vi "pressure system controller v13 MEMStoGO (old) 2015.vi"() -> ()   [LabVIEW 2015]
uses:
  <vilib>/DAQmx/write.llb/DAQmx Write (Digital 1D Bool 1Chan 1Samp).vi
  <vilib>/DAQmx/write.llb/DAQmx Write (Analog DBL 1Chan 1Samp).vi
  <vilib>/DAQmx/read.llb/DAQmx Read (Analog DBL 1Chan 1Samp).vi
  <vilib>/DAQmx/create/channels.llb/DAQmx Create Channel (DO-Digital Output).vi
  <vilib>/DAQmx/miscellaneous.llb/DAQmx Fill In Error Info.vi
  <vilib>/DAQmx/create/channels.llb/DAQmx Create Channel (AI-Voltage-Basic).vi
  <vilib>/DAQmx/configure/timing.llb/DAQmx Timing (Sample Clock).vi
  <vilib>/DAQmx/create/channels.llb/DAQmx Create Channel (AO-Current-Basic).vi
  <vilib>/express/express shared/transition.llb/Dynamic To Waveform Array.vi
  <vilib>/express/express signal manip/GetorSetDDTAttributes/Set DDT Attributes/SetT0.vi
  <vilib>/express/express shared/transition.llb/Waveform Array To Dynamic.vi
  <instrlib>/Keithley 24XX/Public/Data/Read (Single Point).vi
  <vilib>/express/express signal manip/GetorSetDDTAttributes/Set DDT Attributes/Set DDT Properties.xnode
  <vilib>/ptbypt/NI_PtbyPt.lvlib
  <instrlib>/Keithley 24XX/Keithley 24XX.lvlib
  <instrlib>/Agilent E4980/Agilent E4980.lvlib
panel:
  in  "MUX4: Keithley (-)":T1(radio)
  in  "MUX3: Keithley (+)":T1(radio)
  in  "MUX2: LCR (-)":T1(radio)
  in  "MUX1: LCR (+)":T1(radio)
  in  "Write to file":bool=TRUE caption="Enable"
  out "Pressure":dbl
  in  "Turn on (MAKE SURE TURN OFF)":bool=TRUE
  out "Impedance":dbl format="%^#_6e"
  out "Phase (deg)":dbl
  in  "Function (0: Cp-D)":u16(ring)=17 items=["Cp-D", "Cp-Q", "Cp-G", "Cp-Rp", "Cs-D", "Cs-Q", "Cs-Rs", "Lp-D", "Lp-Q", "Lp-G", "Lp-Rp", "Lp-Rdc", "Ls-D", "Ls-Q", "Ls-Rs", "Ls-Rdc", "R-X", "Z-thd", "Z-thr", "G-B", "Y-thd", "Y-thr", "Vdc-Idc"]
  in  "Signal Level (1.0 V)":dbl=1.0
  in  "Averaging Factor (1)":i32=1
  in  "Measurement Time (1: Medium)":u16(ring) items=["Short", "Medium", "Long"]
  in  "Signal Frequency":dbl=10000.0
  out "Resistance (Mohm)":dbl
  out "Current (uA)":sgl
  out "Voltage":sgl
  in  "Loop sample rate (samples per second)":dbl=5.0
  in  "Current duration (s)":dbl=2.0
  out "Time Counter":i32
  in  "Keithley Output (uA)":dbl=1.0
  in  "Compliance (V)":dbl=21.0
  in  "Inject Current":bool
  out "Supply Current":dbl
  in  "Set Point Pressure (mmHg)":dbl min=0.0 max=500.0
  in  "stop":bool
  # "Switch"
  # "Keithley Settings"
  # "Pressure Setup"
  # "LCR Settings"
  # "1KHz for water"
  # "MAX: 500"
  # "10KHz for PBS"
  # "seconds"
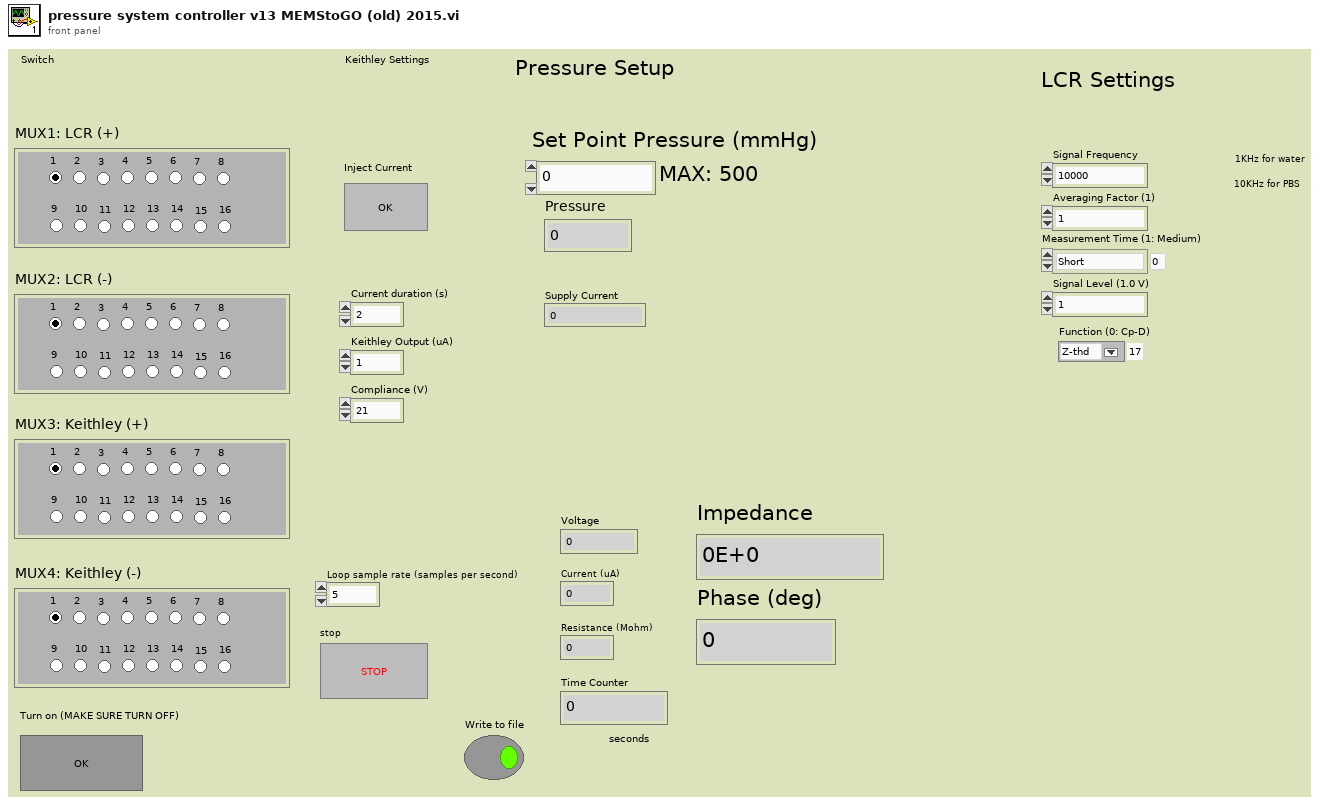
[diagram p1: front panel]
types:
  T1 = enum32{"1", "2", "3", "4", "5", "6", "7", "8", "9", "10", "11", "12", "13", "14", "15", "16"}
  T2 = cluster{"Primary Parameter":dbl, "Secondary Parameter":dbl}
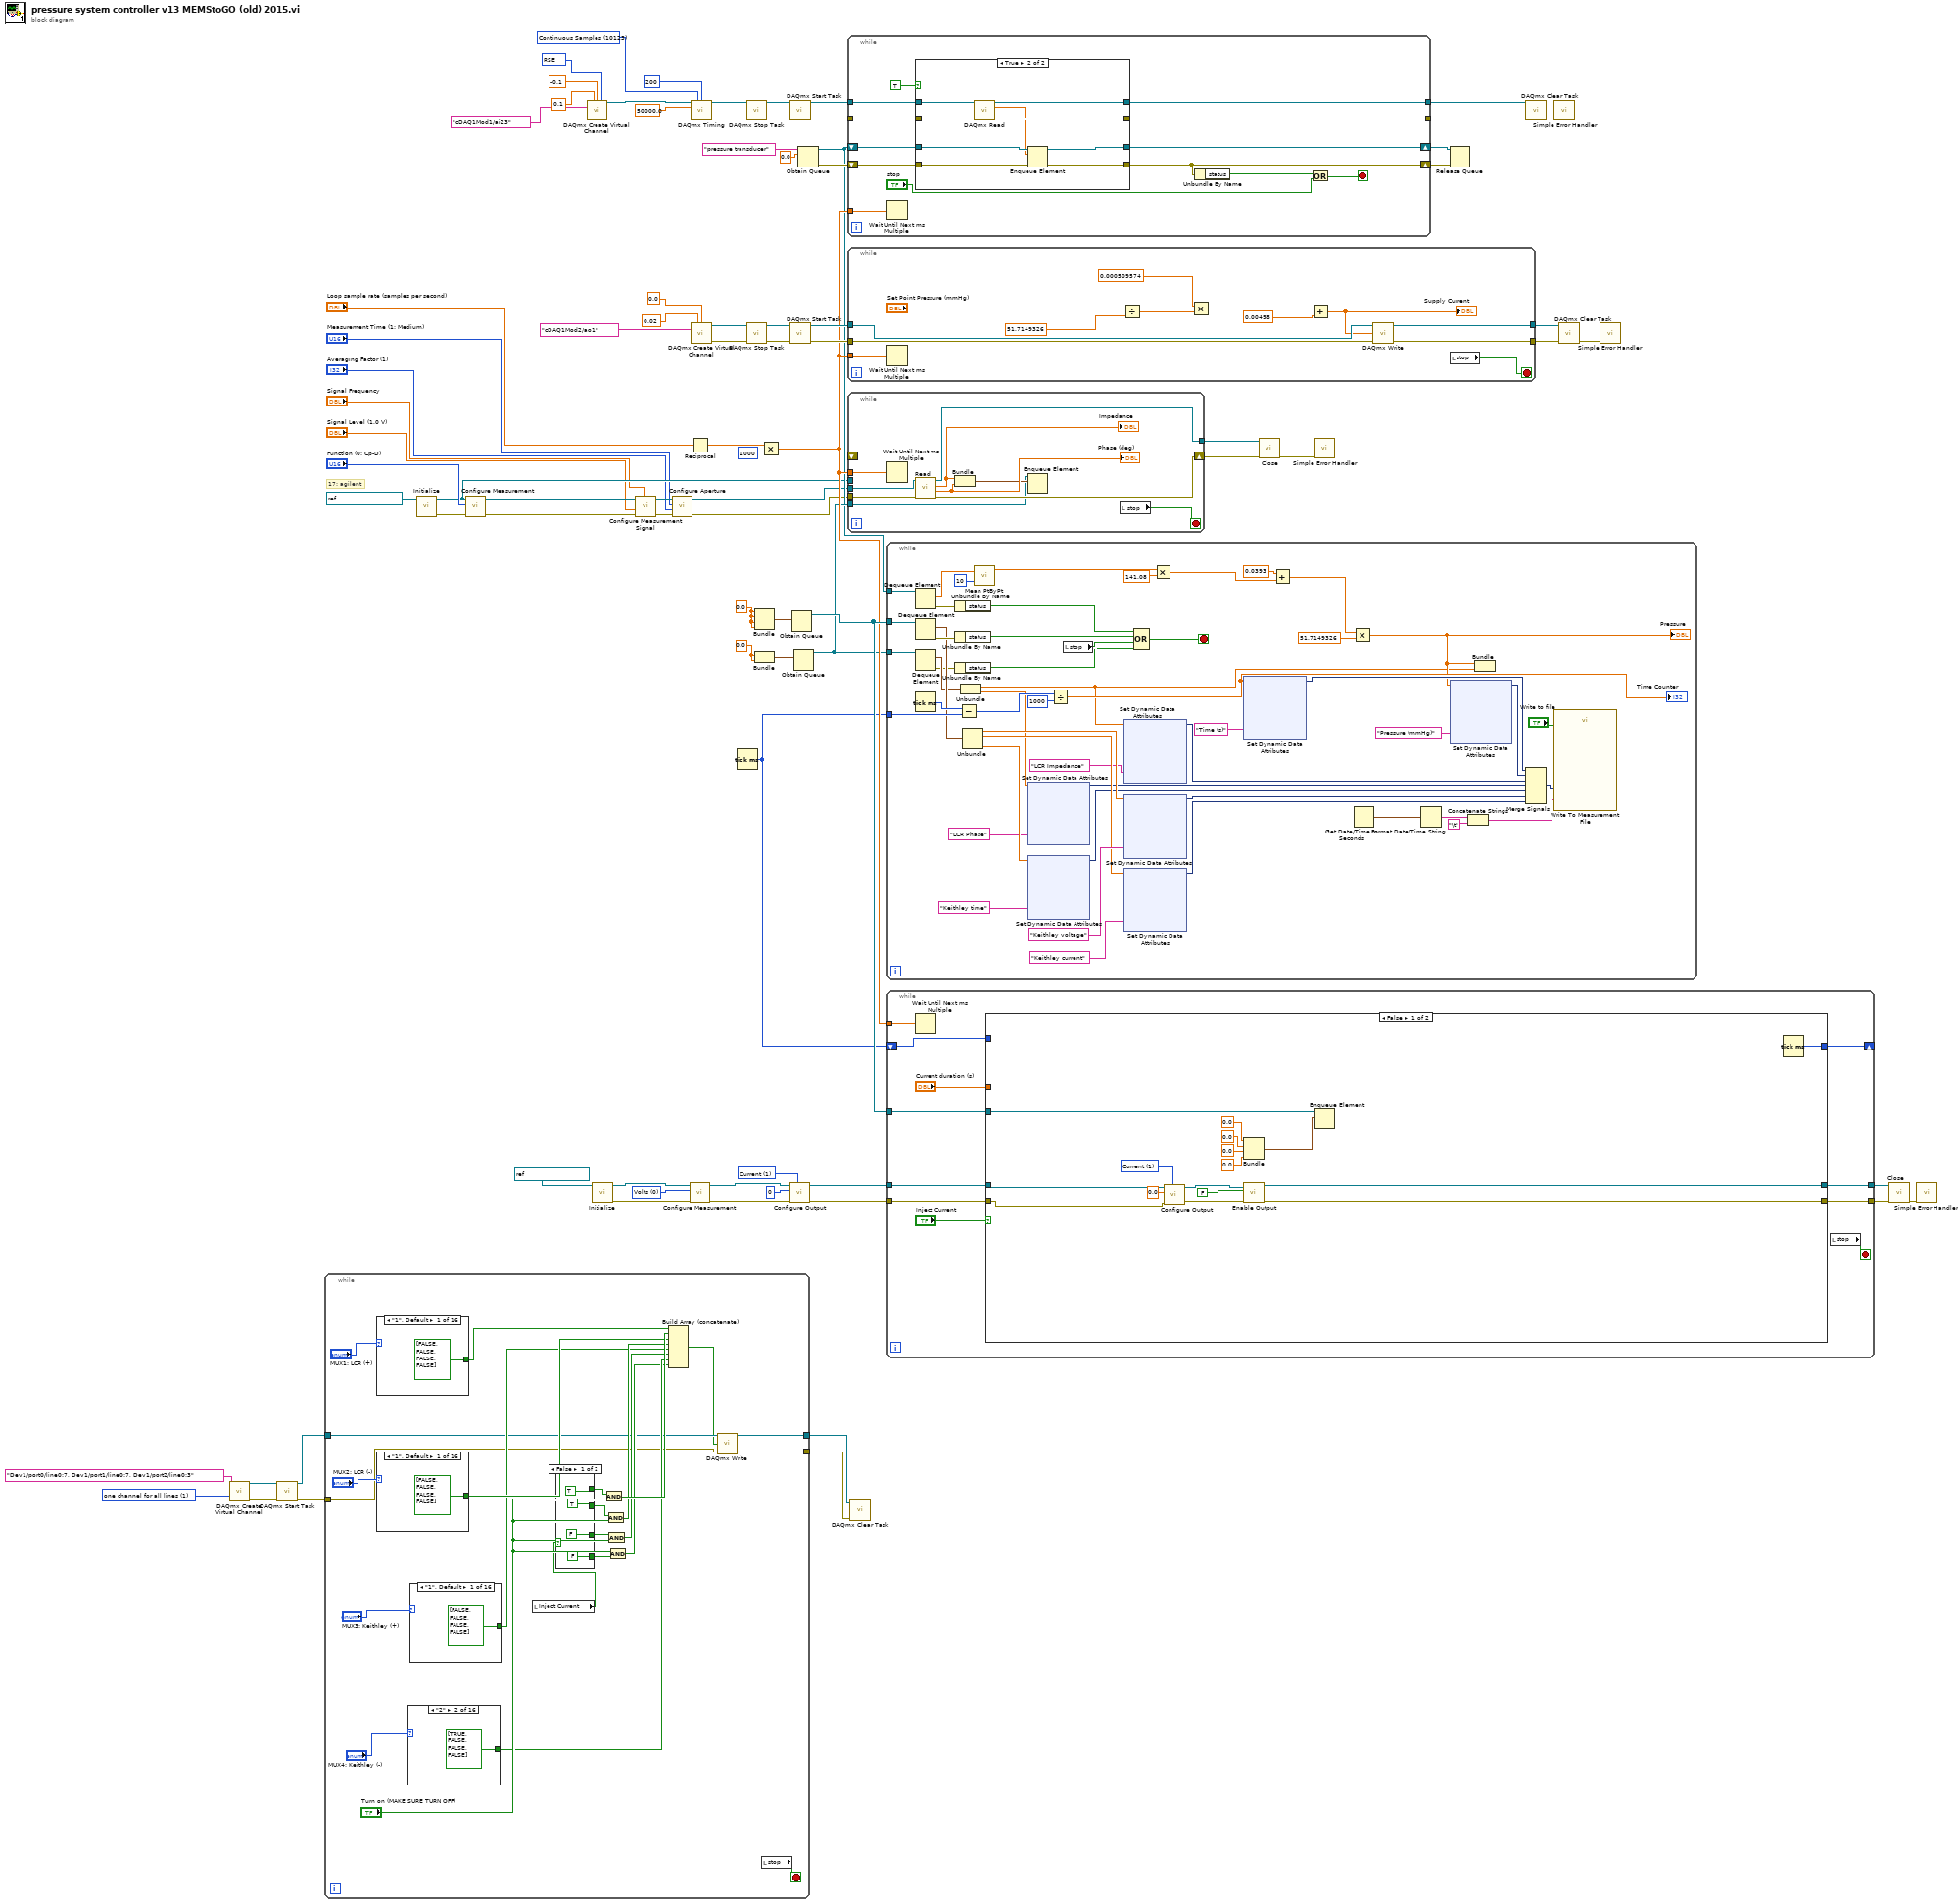
[diagram p0: block diagram]
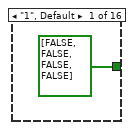
[diagram p2: hidden frame]
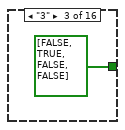
[diagram p3: hidden frame]
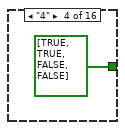
[diagram p4: hidden frame]
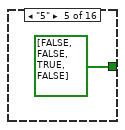
[diagram p5: hidden frame]
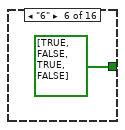
[diagram p6: hidden frame]
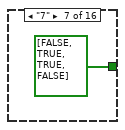
[diagram p7: hidden frame]
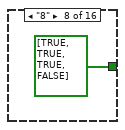
[diagram p8: hidden frame]
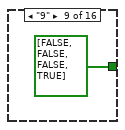
[diagram p9: hidden frame]
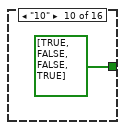
[diagram p10: hidden frame]
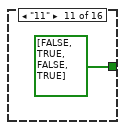
[diagram p11: hidden frame]
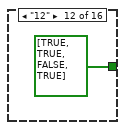
[diagram p12: hidden frame]
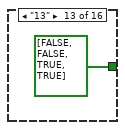
[diagram p13: hidden frame]
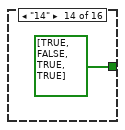
[diagram p14: hidden frame]
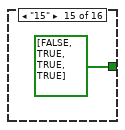
[diagram p15: hidden frame]
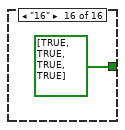
[diagram p16: hidden frame]
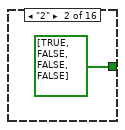
[diagram p17: hidden frame]
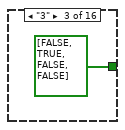
[diagram p18: hidden frame]
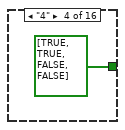
[diagram p19: hidden frame]
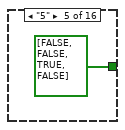
[diagram p20: hidden frame]
diagram:
  w11 = 1 items=["one channel for each line", "one channel for all lines"] ("line grouping")
  w48 = u16 1 items=["Voltage", "Current"] ("Source Mode  (0: Voltage)")
  w54 = u16 0 items=["Volts", "Current", "Resistance"] ("Keithley Measure")
  w33 = sgl 0.0 ("y")
  w42 = sgl 0.0 ("y")
  w82 = 10123 items=["Finite Samples"=10178, "Continuous Samples"=10123, "Hardware Timed Single Point"=12522] ("sample mode")
  w85 = 10083 items=["default"=-1, "RSE"=10083, "NRSE"=10078, "Differential"=10106, "Pseudodifferential"=12529] ("input terminal configuration")
  # "17: agilent"
  n1 = call-poly <vilib>:"DAQmx Create Virtual Channel.vi"("lines"=tag "Dev1/port0/line0:7, Dev1/port1/line0:7, Dev1/port2/line0:3", "line grouping"=w11) -> ("task out"=w9:refnum<k21>, "error out"=w10:errorcluster)  [unwired: 12 in]
  n2 = call <vilib>:"DAQmx Start Task.vi"("task/channels in"=w9, "error in"=w10) -> ("task out"=w7:refnum<k21>, "error out"=w5:errorcluster)  [unwired: 12 in]
  n3 = while {
    tunnel: w7 -> [w91]
    tunnel: [w90] -> w6
    tunnel: w5 -> [w89]
    tunnel: [w88] -> w4
    stop <- w108 stop-if-true
    n4 = case shown="\"1\", Default" "MUX1: LCR (+)" {
      tunnel: [bool[] [FALSE, FALSE, FALSE, FALSE] bool[] [TRUE, FALSE, FALSE, FALSE] bool[] [FALSE, TRUE, FALSE, FALSE] bool[] [TRUE, TRUE, FALSE, FALSE] bool[] [FALSE, FALSE, TRUE, FALSE] bool[] [TRUE, FALSE, TRUE, FALSE] bool[] [FALSE, TRUE, TRUE, FALSE] bool[] [TRUE, TRUE, TRUE, FALSE] bool[] [FALSE, FALSE, FALSE, TRUE] bool[] [TRUE, FALSE, FALSE, TRUE] bool[] [FALSE, TRUE, FALSE, TRUE] bool[] [TRUE, TRUE, FALSE, TRUE] bool[] [FALSE, FALSE, TRUE, TRUE] bool[] [TRUE, FALSE, TRUE, TRUE] bool[] [FALSE, TRUE, TRUE, TRUE] bool[] [TRUE, TRUE, TRUE, TRUE]] -> w99
      frame "1", Default {
      }
      frame "2" {
      }
      frame "3" {
      }
      frame "4" {
      }
      frame "5" {
      }
      frame "6" {
      }
      frame "7" {
      }
      frame "8" {
      }
      frame "9" {
      }
      frame "10" {
      }
      frame "11" {
      }
      frame "12" {
      }
      frame "13" {
      }
      frame "14" {
      }
      frame "15" {
      }
      frame "16" {
      }
    }
    n5 = case shown="\"1\", Default" "MUX2: LCR (-)" {
      tunnel: [bool[] [FALSE, FALSE, FALSE, FALSE] bool[] [TRUE, FALSE, FALSE, FALSE] bool[] [FALSE, TRUE, FALSE, FALSE] bool[] [TRUE, TRUE, FALSE, FALSE] bool[] [FALSE, FALSE, TRUE, FALSE] bool[] [TRUE, FALSE, TRUE, FALSE] bool[] [FALSE, TRUE, TRUE, FALSE] bool[] [TRUE, TRUE, TRUE, FALSE] bool[] [FALSE, FALSE, FALSE, TRUE] bool[] [TRUE, FALSE, FALSE, TRUE] bool[] [FALSE, TRUE, FALSE, TRUE] bool[] [TRUE, TRUE, FALSE, TRUE] bool[] [FALSE, FALSE, TRUE, TRUE] bool[] [TRUE, FALSE, TRUE, TRUE] bool[] [FALSE, TRUE, TRUE, TRUE] bool[] [TRUE, TRUE, TRUE, TRUE]] -> w97
      frame "1", Default {
      }
      frame "2" {
      }
      frame "3" {
      }
      frame "4" {
      }
      frame "5" {
      }
      frame "6" {
      }
      frame "7" {
      }
      frame "8" {
      }
      frame "9" {
      }
      frame "10" {
      }
      frame "11" {
      }
      frame "12" {
      }
      frame "13" {
      }
      frame "14" {
      }
      frame "15" {
      }
      frame "16" {
      }
    }
    n6 = case shown="\"2\"" "MUX4: Keithley (-)" {
      tunnel: [bool[] [FALSE, FALSE, FALSE, FALSE] bool[] [TRUE, FALSE, FALSE, FALSE] bool[] [FALSE, TRUE, FALSE, FALSE] bool[] [TRUE, TRUE, FALSE, FALSE] bool[] [FALSE, FALSE, TRUE, FALSE] bool[] [TRUE, FALSE, TRUE, FALSE] bool[] [FALSE, TRUE, TRUE, FALSE] bool[] [TRUE, TRUE, TRUE, FALSE] bool[] [FALSE, FALSE, FALSE, TRUE] bool[] [TRUE, FALSE, FALSE, TRUE] bool[] [FALSE, TRUE, FALSE, TRUE] bool[] [TRUE, TRUE, FALSE, TRUE] bool[] [FALSE, FALSE, TRUE, TRUE] bool[] [TRUE, FALSE, TRUE, TRUE] bool[] [FALSE, TRUE, TRUE, TRUE] bool[] [TRUE, TRUE, TRUE, TRUE]] -> w93
      frame "1", Default {
      }
      frame "2" {
      }
      frame "3" {
      }
      frame "4" {
      }
      frame "5" {
      }
      frame "6" {
      }
      frame "7" {
      }
      frame "8" {
      }
      frame "9" {
      }
      frame "10" {
      }
      frame "11" {
      }
      frame "12" {
      }
      frame "13" {
      }
      frame "14" {
      }
      frame "15" {
      }
      frame "16" {
      }
    }
    n7 = case shown="\"1\", Default" "MUX3: Keithley (+)" {
      tunnel: [bool[] [FALSE, FALSE, FALSE, FALSE] bool[] [TRUE, FALSE, FALSE, FALSE] bool[] [FALSE, TRUE, FALSE, FALSE] bool[] [TRUE, TRUE, FALSE, FALSE] bool[] [FALSE, FALSE, TRUE, FALSE] bool[] [TRUE, FALSE, TRUE, FALSE] bool[] [FALSE, TRUE, TRUE, FALSE] bool[] [TRUE, TRUE, TRUE, FALSE] bool[] [FALSE, FALSE, FALSE, TRUE] bool[] [TRUE, FALSE, FALSE, TRUE] bool[] [FALSE, TRUE, FALSE, TRUE] bool[] [TRUE, TRUE, FALSE, TRUE] bool[] [FALSE, FALSE, TRUE, TRUE] bool[] [TRUE, FALSE, TRUE, TRUE] bool[] [FALSE, TRUE, TRUE, TRUE] bool[] [TRUE, TRUE, TRUE, TRUE]] -> w95
      frame "1", Default {
      }
      frame "2" {
      }
      frame "3" {
      }
      frame "4" {
      }
      frame "5" {
      }
      frame "6" {
      }
      frame "7" {
      }
      frame "8" {
      }
      frame "9" {
      }
      frame "10" {
      }
      frame "11" {
      }
      frame "12" {
      }
      frame "13" {
      }
      frame "14" {
      }
      frame "15" {
      }
      frame "16" {
      }
    }
    n8 = local read "Inject Current"() -> (w86:bool)
    n9 = case shown="False" w86 {
      tunnel: [TRUE FALSE] -> w103
      tunnel: [TRUE FALSE] -> w102
      tunnel: [FALSE TRUE] -> w101
      tunnel: [FALSE TRUE] -> w100
      frame False {
      }
      frame True {
      }
    }
    n10 = And(x=w103, y="Turn on (MAKE SURE TURN OFF)") -> (x .and. y?=w98:bool)
    n11 = And(x=w102, y="Turn on (MAKE SURE TURN OFF)") -> (x .and. y?=w96:bool)
    n12 = And(x=w101, y="Turn on (MAKE SURE TURN OFF)") -> (x .and. y?=w94:bool)
    n13 = And(x="Turn on (MAKE SURE TURN OFF)", y=w100) -> (x .and. y?=w92:bool)
    n14 = Build Array (concatenate)(w99, w98, w97, w96, w95, w94, w93, w92) -> (w87:bool[])
    n15 = call-poly <vilib>:"DAQmx Write.vi"("task/channels in"=w91, "data"=w87, "error in"=w89) -> ("task out"=w90:refnum<k21>, "error out"=w88:errorcluster)  [unwired: 10 in, 1 out]
    n16 = local read "stop"() -> (w108:bool)
  }
  n17 = call <instrlib>:"Initialize.vi"("VISA resource name"=refnum<visa-resource-name> "GPIB0::16::INSTR") -> ("error out"=w24:errorcluster, "VISA resource name out"=w23:refnum<visa-resource-name>)  [unwired: 9 in]
  n18 = call <instrlib>:"Configure Measurement.vi"("error in (no error)"=w24, "Function (0: Cp-D)"="Function (0: Cp-D)", "VISA resource name"=w23) -> ("error out"=w22:errorcluster, "VISA resource name out"=w21:refnum<visa-resource-name>)  [unwired: 7 in]
  n19 = call-poly <vilib>:"DAQmx Create Virtual Channel.vi"("maximum value"=0.1, "minimum value"=-0.1, "input terminal configuration"=w85, "physical channels"=tag "cDAQ1Mod1/ai23") -> ("task out"=w79:refnum<k21>, "error out"=w78:errorcluster)  [unwired: 10 in]
  n20 = call <instrlib>:"Initialize.vi"("VISA resource name"=refnum<visa-resource-name> "GPIB0::24::INSTR") -> ("error out"=w52:errorcluster, "VISA resource name out"=w53:refnum<visa-resource-name>)  [unwired: 9 in]
  n21 = call <instrlib>:"Configure Measurement Signal.vi"("Signal Frequency (1000 Hz)"="Signal Frequency", "error in (no error)"=w22, "Signal Level (1.0 V)"="Signal Level (1.0 V)", "VISA resource name"=w21) -> ("error out"=w18:errorcluster, "VISA resource name out"=w17:refnum<visa-resource-name>)  [unwired: 6 in]
  n22 = call <instrlib>:"Configure Aperture.vi"("error in (no error)"=w18, "Averaging Factor (1)"="Averaging Factor (1)", "Measurement Time (1: Medium)"="Measurement Time (1: Medium)", "VISA resource name"=w17) -> ("error out"=w14:errorcluster, "VISA resource name out"=w13:refnum<visa-resource-name>)  [unwired: 6 in]
  n23 = call <instrlib>:"Configure Measurement.vi"("error in (no error)"=w52, "Function (0: Volts)"=w54, "VISA resource name"=w53) -> ("error out"=w50:errorcluster, "VISA resource name out"=w51:refnum<visa-resource-name>)  [unwired: 7 in]
  n24 = Reciprocal(x="Loop sample rate (samples per second)") -> (1/x=w39:dbl)
  n25 = call-poly <vilib>:"DAQmx Timing.vi"("task/channels in"=w79, "sample mode"=w82, "samples per channel"=200, "rate"=50000.0, "error in"=w78) -> ("task out"=w77:refnum<k21>, "error out"=w76:errorcluster)  [unwired: 9 in]
  n26 = call-poly <vilib>:"DAQmx Create Virtual Channel.vi"("maximum value"=0.02, "minimum value"=0.0, "physical channels"=tag "cDAQ1Mod2/ao1") -> ("task out"=w60:refnum<k21>, "error out"=w59:errorcluster)  [unwired: 11 in]
  n27 = Tick Count (ms)() -> (millisecond timer value=w3:u32)
  n28 = call <vilib>:"DAQmx Stop Task.vi"("task/channels in"=w77, "error in"=w76) -> ("task out"=w75:refnum<k21>, "error out"=w74:errorcluster)  [unwired: 12 in]
  n29 = call <vilib>:"DAQmx Stop Task.vi"("task/channels in"=w60, "error in"=w59) -> ("task out"=w62:refnum<k21>, "error out"=w61:errorcluster)  [unwired: 12 in]
  n30 = Bundle("y"=w42, "y"=w42, "y"=w42, "y"=w42) -> (w41:cluster{"y":sgl, "y":sgl, "y":sgl, "y":sgl})  [unwired: 1 in]
  n31 = Bundle("y"=w33, "y"=w33) -> (w32:cluster{"y":sgl, "y":sgl})  [unwired: 1 in]
  n32 = Multiply(x=w39, y=1000) -> (x*y=w34:dbl)
  n33 = call <instrlib>:"Configure Output.vi"("Source Mode  (0: Voltage)"=w48, "error in (no error)"=w50, "Output Level (0)"=0, "VISA resource name"=w51) -> ("error out"=w46:errorcluster, "VISA resource name out"=w47:refnum<visa-resource-name>)  [unwired: 6 in]
  n34 = call <vilib>:"DAQmx Start Task.vi"("task/channels in"=w75, "error in"=w74) -> ("task out"=w69:refnum<k21>, "error out"=w68:errorcluster)  [unwired: 12 in]
  n35 = call <vilib>:"DAQmx Start Task.vi"("task/channels in"=w62, "error in"=w61) -> ("task out"=w58:refnum<k21>, "error out"=w57:errorcluster)  [unwired: 12 in]
  n36 = Obtain Queue(element data type=w41) -> (queue out=w45:refnum<queue>)  [unwired: 4 in, 2 out]
  n37 = Obtain Queue(element data type=w32) -> (queue out=w31:refnum<queue>)  [unwired: 4 in, 2 out]
  n38 = Obtain Queue(name (unnamed)="pressure transducer", element data type=sgl 0.0 ("kvoltage")) -> (queue out=w26:refnum<queue>, error out=w73:errorcluster)  [unwired: 3 in, 1 out]
  n39 = while {
    shift-right: [w191] -> w71
    shift-left: w73 -> [w193]
    tunnel: w69 -> [w189]
    tunnel: w68 -> [w188]
    tunnel: [w187] -> w67
    tunnel: [w186] -> w66
    shift-right: [w192] -> w72
    shift-left: w26 -> [w194]
    tunnel: w34 -> [w183]
    stop <- w185 stop-if-true
    n40 = Wait Until Next ms Multiple(millisecond multiple=w183) -> ()  [unwired: 1 out]
    n41 = case shown="True" TRUE {
      tunnel: w194 -> [w198 w207]
      tunnel: w193 -> [w197 w206]
      tunnel: [w198 w205] -> w192
      tunnel: [w197 w204] -> w191
      tunnel: w189 -> [w196 w203]
      tunnel: w188 -> [w195 w202]
      tunnel: [w196 w201] -> w187
      tunnel: [w195 w200] -> w186
      frame False {
      }
      frame True {
        n42 = call-poly <vilib>:"DAQmx Read.vi"("task/channels in"=w203, "error in"=w202) -> ("task out"=w201:refnum<k21>, "data"=w199:dbl, "error out"=w200:errorcluster)  [unwired: 11 in]
        n43 = Enqueue Element(queue=w207, element=w199, error in (no error)=w206) -> (queue out=w205:refnum<queue>, error out=w204:errorcluster)  [unwired: 1 in, 1 out]
      }
    }
    n44 = Unbundle By Name(w191) -> ("status"=w190:bool)
    n45 = Or(x=w190, y="stop") -> (x .or. y?=w185:bool)
  }
  n46 = while {
    tunnel: w58 -> [w219]
    tunnel: w57 -> [w218]
    tunnel: [w217] -> w56
    tunnel: [w216] -> w55
    tunnel: w34 -> [w214]
    stop <- w215 stop-if-true
    n47 = Wait Until Next ms Multiple(millisecond multiple=w214) -> ()  [unwired: 1 out]
    n48 = Divide(x="Set Point Pressure (mmHg)", y=51.7149326) -> (x/y=w212:dbl)
    n49 = Multiply(x=0.000509574, y=w212) -> (x*y=w210:dbl)
    n50 = Add(x=w210, y=0.00498) -> (x+y=w208:dbl)
    "Supply Current" <- w208
    n51 = call-poly <vilib>:"DAQmx Write.vi"("task/channels in"=w219, "data"=w208, "error in"=w218) -> ("task out"=w217:refnum<k21>, "error out"=w216:errorcluster)  [unwired: 10 in, 1 out]
    n52 = local read "stop"() -> (w215:bool)
  }
  n53 = while {
    shift-right: [w230] -> w36
    shift-left: _ -> [_]
    tunnel: w23 -> [_]
    tunnel: [w229] -> w35
    tunnel: w34 -> [w228]
    tunnel: w31 -> [w224]
    tunnel: w14 -> [w222]
    tunnel: w13 -> [w221]
    stop <- w223 stop-if-true
    n54 = Wait Until Next ms Multiple(millisecond multiple=w228) -> ()  [unwired: 1 out]
    n55 = call <instrlib>:"Read.vi"("error in (no error)"=w222, "VISA resource name"=w221) -> ("error out"=w230:errorcluster, "Secondary Parameter"=w227:dbl, "Primary Parameter"=w226:dbl, "VISA resource name out"=w229:refnum<visa-resource-name>)  [unwired: 6 in]
    "Phase (deg)" <- w227
    "Impedance" <- w226
    n56 = Bundle("Primary Parameter"=w226, "Secondary Parameter"=w227) -> (w225:T2)  [unwired: 1 in]
    n57 = Enqueue Element(queue=w224, element=w225) -> ()  [unwired: 2 in, 3 out]
    n58 = local read "stop"() -> (w223:bool)
  }
  n59 = call <vilib>:"DAQmx Clear Task.vi"("task in"=w6, "error in"=w4) -> ()  [unwired: 13 in, 1 out]
  n60 = while {
    tunnel: w26 -> [w281]
    tunnel: w3 -> [w269]
    tunnel: w45 -> [w265]
    tunnel: w31 -> [w250]
    stop <- w261 stop-if-true
    n61 = Dequeue Element(queue=w281) -> (element=w243:sgl, error out=w282:errorcluster)  [unwired: 2 in, 2 out]
    n62 = Dequeue Element(queue=w265) -> (element=w260:cluster{"y":sgl, "y":sgl, "y":sgl, "y":sgl}, error out=w264:errorcluster)  [unwired: 2 in, 2 out]
    n63 = Dequeue Element(queue=w250) -> (element=w249:cluster{"y":sgl, "y":sgl}, error out=w245:errorcluster)  [unwired: 2 in, 2 out]
    n64 = Tick Count (ms)() -> (millisecond timer value=w272:u32)
    n65 = Unbundle By Name(w282) -> ("status"=w263:bool)
    n66 = Unbundle By Name(w264) -> ("status"=w262:bool)
    n67 = Unbundle By Name(w245) -> ("status"=w244:bool)
    n68 = Subtract(x=w272, y=w269) -> (x-y=w270:u32)
    n69 = Unbundle(w249) -> ("y"=w246:sgl, "y"=w248:sgl)
    n70 = Unbundle(w260) -> ("y"=w255:sgl, "y"=w254:sgl, "y"=w256:sgl)  [unwired: 1 out]
    n71 = call <vilib>:"Mean PtByPt.vi"("x"=w243, "sample length"=10) -> ("mean"=w236:dbl)  [unwired: 2 in, 1 out]
    n72 = xnode "Set Dynamic Data Attributes"("Signal Name"="LCR Phase", "Signals In"=w248) -> ("Signals Out"=w240:dynamicdata)  [unwired: 2 in, 1 out]
    n73 = xnode "Set Dynamic Data Attributes"("Signal Name"="Keithley time", "Signals In"=w256) -> ("Signals Out"=w239:dynamicdata)  [unwired: 2 in, 1 out]
    n74 = Divide(x=w270, y=1000) -> (x/y=w267:dbl)
    "Time Counter" <- w267
    n75 = local read "stop"() -> (w253:bool)
    n76 = xnode "Set Dynamic Data Attributes"("Signal Name"="LCR Impedance", "Signals In"=w246) -> ("Signals Out"=w241:dynamicdata)  [unwired: 2 in, 1 out]
    n77 = xnode "Set Dynamic Data Attributes"("Signal Name"="Keithley voltage", "Signals In"=w255) -> ("Signals Out"=w238:dynamicdata)  [unwired: 2 in, 1 out]
    n78 = xnode "Set Dynamic Data Attributes"("Signal Name"="Keithley current", "Signals In"=w254) -> ("Signals Out"=w237:dynamicdata)  [unwired: 2 in, 1 out]
    n79 = Compound Arithmetic op=OR(w263, w262, w253, w244) -> (w261:bool)
    n80 = Multiply(x=w236, y=141.08) -> (x*y=w234:dbl)
    n81 = xnode "Set Dynamic Data Attributes"("Signal Name"="Time (s)", "Signals In"=w267) -> ("Signals Out"=w266:dynamicdata)  [unwired: 2 in, 1 out]
    n82 = Add(x=0.0393, y=w234) -> (x+y=w232:dbl)
    n83 = Multiply(x=w232, y=51.7149326) -> (x*y=w247:dbl)
    "Pressure" <- w247
    n84 = Get Date/Time In Seconds() -> (seconds since 1Jan1904=w276:timestamp)
    n85 = Format Date/Time String(seconds (now)=w276) -> (date/time string=w277:string)  [unwired: 2 in]
    n86 = xnode "Set Dynamic Data Attributes"("Signal Name"="Pressure (mmHg)", "Signals In"=w247) -> ("Signals Out"=w274:dynamicdata)  [unwired: 2 in, 1 out]
    n87 = Concatenate Strings(w277, "\t") -> (w275:string)
    n88 = Bundle(w247, "y"=w246) -> ()  [unwired: 1 in, 1 out]
    n89 = Merge Signals(w266, w274, w241, w240, w239, w238, w237) -> (w273:dynamicdata)
    n90 = call "Write To Measurement File"("Signals"=w273, "Enable"="Write to file", "Comment"=w275) -> ()  [unwired: 14 in, 3 out]
  }
  n91 = while {
    tunnel: w47 -> [w391]
    tunnel: w46 -> [w390]
    tunnel: w45 -> [w387]
    tunnel: [w382] -> w44
    tunnel: [w381] -> w43
    shift-right: [w385] -> _
    shift-left: w3 -> [w384]
    tunnel: w34 -> [w383]
    stop <- w388 stop-if-true
    n92 = Wait Until Next ms Multiple(millisecond multiple=w383) -> ()  [unwired: 1 out]
    n93 = case shown="False" "Inject Current" {
      selector: "Inject Current" -> [_ w414]
      tunnel: w391 -> [w397 w438]
      tunnel: w390 -> [w396 w437]
      tunnel: w387 -> [w405 w430]
      tunnel: "Current duration (s)" -> [_ w428]
      tunnel: [w407 w422] -> w382
      tunnel: [w406 w421] -> w381
      tunnel: [w399 w419] -> w385
      tunnel: w384 -> [_ w419]
      frame False {
        w392 = u16 1 items=["Voltage", "Current"] ("Source Mode  (0: Voltage)")
        n94 = call <instrlib>:"Configure Output.vi"("Source Mode  (0: Voltage)"=w392, "error in (no error)"=w396, "Output Level (0)"=0.0, "VISA resource name"=w397) -> ("error out"=w394:errorcluster, "VISA resource name out"=w395:refnum<visa-resource-name>)  [unwired: 6 in]
        n95 = Bundle("y"=sgl 0.0, "y"=sgl 0.0, "y"=sgl 0.0, "y"=sgl 0.0) -> (w404:cluster{"y":sgl, "y":sgl, "y":sgl, "y":sgl})  [unwired: 1 in]
        n96 = call <instrlib>:"Enable Output.vi"("error in (no error)"=w394, "Enable Output (T: Enable)"=FALSE, "VISA resource name"=w395) -> ("error out"=w406:errorcluster, "VISA resource name out"=w407:refnum<visa-resource-name>)  [unwired: 7 in]
        n97 = Enqueue Element(queue=w405, element=w404) -> ()  [unwired: 2 in, 3 out]
        n98 = Tick Count (ms)() -> (millisecond timer value=w399:u32)
      }
      frame True {
        w411 = u16 1 items=["Voltage", "Current"] ("Source Mode  (0: Voltage)")
        n99 = Tick Count (ms)() -> (millisecond timer value=w420:u32)
        n100 = Subtract(x=w420, y=w419) -> (x-y=w415:u32)
        n101 = call <instrlib>:"Enable Output.vi"("error in (no error)"=w437, "Enable Output (T: Enable)"=w414, "VISA resource name"=w438) -> ("error out"=w412:errorcluster, "VISA resource name out"=w413:refnum<visa-resource-name>)  [unwired: 7 in]
        n102 = Divide(x=w415, y=1000) -> (x/y=w425:dbl)
        n103 = Multiply(x="Keithley Output (uA)", y=1e-06) -> (x*y=w416:dbl)
        n104 = Greater Or Equal?(x=w425, y=w428) -> (x >= y?=w426:bool)
        n105 = Not(x=w426) -> (.not. x?=w427:bool)
        n106 = local write "Inject Current"(w427) -> ()
        n107 = call <instrlib>:"Configure Output.vi"("Source Mode  (0: Voltage)"=w411, "error in (no error)"=w412, "Compliance  Level (0.1)"="Compliance (V)", "Output Level (0)"=w416, "VISA resource name"=w413) -> ("error out"=w408:errorcluster, "VISA resource name out"=w409:refnum<visa-resource-name>)  [unwired: 5 in]
        n108 = call-poly <instrlib>:"Read.vi"("VISA resource name"=w409, "error in (no error)"=w408) -> ("Voltage"=w424:sgl, "VISA resource name out"=w422:refnum<visa-resource-name>, "Current"=w436:sgl, "Resistance"=w434:sgl, "error out"=w421:errorcluster)  [unwired: 7 in, 2 out]
        "Voltage" <- w424
        n109 = Multiply(x=w434, y=1e-06) -> (x*y=w432:dbl)
        "Resistance (Mohm)" <- w432
        n110 = Multiply(x=w436, y=sgl 1000000.0) -> (x*y=w423:sgl)
        "Current (uA)" <- w423
        n111 = Bundle("Voltage"=w424, w423, w432, w425) -> (w431:cluster{"Voltage":sgl, sgl, dbl, dbl})  [unwired: 1 in]
        n112 = Enqueue Element(queue=w430, element=w431) -> ()  [unwired: 2 in, 3 out]
      }
    }
    n113 = local read "stop"() -> (w388:bool)
  }
  n114 = call <instrlib>:"Close.vi"("error in (no error)"=w36, "VISA resource name"=w35) -> ("error out"=w29:errorcluster)  [unwired: 9 in]
  n115 = call <vilib>:"Simple Error Handler.vi"("error in (no error)"=w29) -> ()  [unwired: 4 in, 5 out]
  n116 = Release Queue(queue=w72, error in (no error)=w71) -> ()  [unwired: 1 in, 3 out]
  n117 = call <vilib>:"DAQmx Clear Task.vi"("task in"=w67, "error in"=w66) -> ("error out"=w28:errorcluster)  [unwired: 13 in]
  n118 = call <vilib>:"Simple Error Handler.vi"("error in (no error)"=w28) -> ()  [unwired: 4 in, 5 out]
  n119 = call <vilib>:"DAQmx Clear Task.vi"("task in"=w56, "error in"=w55) -> ("error out"=w27:errorcluster)  [unwired: 13 in]
  n120 = call <vilib>:"Simple Error Handler.vi"("error in (no error)"=w27) -> ()  [unwired: 4 in, 5 out]
  n121 = call <instrlib>:"Close.vi"("error in (no error)"=w43, "VISA resource name"=w44) -> ("error out"=w30:errorcluster)  [unwired: 9 in]
  n122 = call <vilib>:"Simple Error Handler.vi"("error in (no error)"=w30) -> ()  [unwired: 4 in, 5 out]
